vi "Cmd.ReadExecuteCondition.vi"(6 "Timeout [ms] (1000)":i32=1000, 8 "error in":errorcluster, 11 "cID in":refnum<k5>) -> (0 "error out":errorcluster, 2 "ExecConNo":i32, 3 "cID out":refnum<k5>)   [LabVIEW 2016]
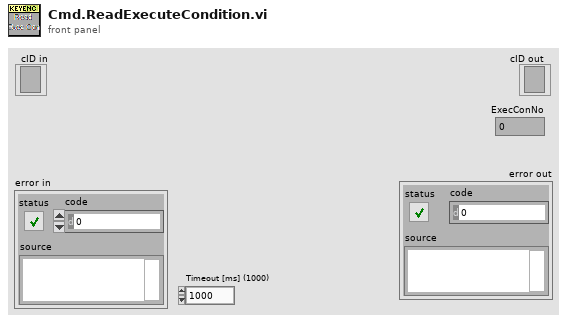
[diagram p1: front panel]
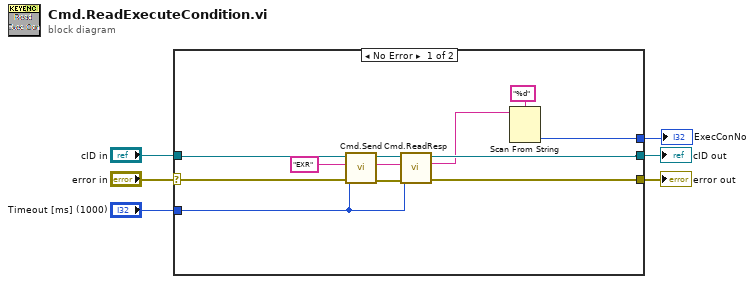
[diagram p0: block diagram]
diagram:
  n1 = case shown="No Error" "error in" {
    selector: "error in" -> [w16 w18]
    tunnel: "Timeout [ms] (1000)" -> [w13 _]
    tunnel: "cID in" -> [w17 w19]
    tunnel: [w12 w19] -> w3
    tunnel: [w11 w18] -> w2
    tunnel: [w7 _] -> w1
    frame No Error {
      w10 = "EXR"
      n2 = call "Cmd.Send.vi"("error in (no error)"=w16, "Timeout [ms] (1000)"=w13, "Command"=w10, "connection ID"=w17) -> ("error out"=w14:errorcluster, "connection ID out"=w15:refnum<k5>)  [unwired: 6 in]
      n3 = call "Cmd.ReadResp.vi"("error in (no error)"=w14, "Timeout [ms] (1000)"=w13, "Request"=w10, "connection ID"=w15) -> ("error out"=w11:errorcluster, "ResponseParameters"=w9:string, "connection ID out"=w12:refnum<k5>)  [unwired: 5 in]
      n4 = Scan From String(format string="%d", input string=w9) -> (output 1=w7:i32)  [unwired: 3 in, 3 out]
    }
    frame Error {
    }
  }
  "cID out" <- w3
  "error out" <- w2
  "ExecConNo" <- w1
